vi "I2C WriteRead Data.vi"(5 "Address":T2 format="%02x", 6 "NoStop (F)":bool, 7 "I2C #":T1=-1, 8 "error in (no error)":errorcluster, 9 "Len":u8, 10 "Write Data":string, 11 "Session in":refnum<class "Session.lvclass">) -> (0 "error out":errorcluster, 1 "Read Data":string, 3 "Session out":refnum<class "Session.lvclass">)   [LabVIEW 2020, in "CTI.lvlib" / "Session.lvclass"]
uses:
  Session.lvclass
  I2C Address.ctl
  I2C Number.ctl
  DeviceComms/DeviceComms.lvclass
  CTI.lvlib
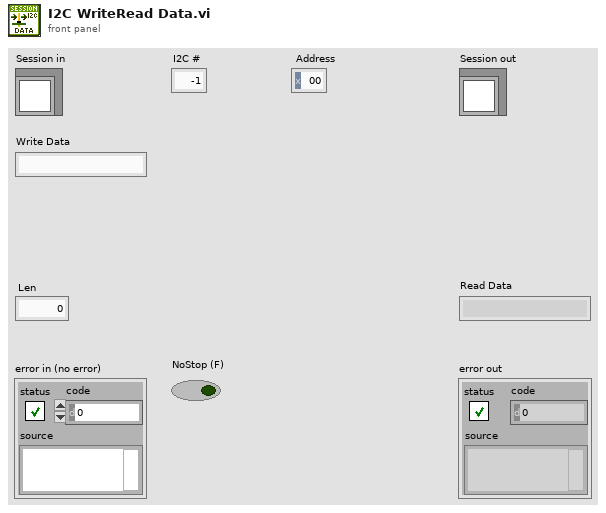
[diagram p1: front panel]
types:
  T1 = typedef "CTI.lvlib/I2C Number.ctl" = i8
  T2 = typedef "CTI.lvlib/I2C Address.ctl" = u8
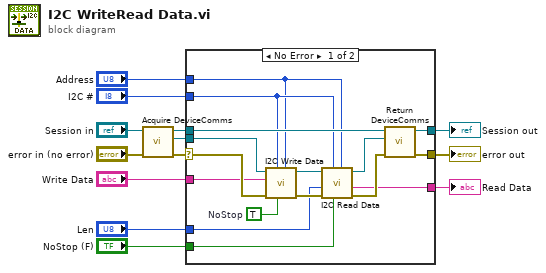
[diagram p0: block diagram]
diagram:
  n1 = call "Acquire DeviceComms.vi"("error in (no error)"="error in (no error)", "Session in"="Session in") -> ("error out"=w12:errorcluster, "DeviceComms"=w11:refnum<class "DeviceComms.lvclass">, "Session out"=w13:refnum<class "Session.lvclass">)  [unwired: 7 in]
  n2 = case shown="No Error" w12 {
    selector: w12 -> [w28 w31]
    tunnel: w13 -> [w27 w30]
    tunnel: w11 -> [w29 _]
    tunnel: [w25 w30] -> w2
    tunnel: [w24 w31] -> w3
    tunnel: "I2C #" -> [w19 _]
    tunnel: "Write Data" -> [w23 _]
    tunnel: "Address" -> [w18 _]
    tunnel: "Len" -> [w17 _]
    tunnel: "NoStop (F)" -> [w16 _]
    tunnel: [w14 _] -> w1
    frame No Error {
      w15 = TRUE  # NoStop
      n3 = call-dynamic "I2C Write Data.vi"("Address"=w18, "NoStop (F)"=w15, "I2C #"=w19, "error in (no error)"=w28, "Data"=w23, "DeviceComms in"=w29) -> ("error out"=w26:errorcluster, "DeviceComms out"=w21:refnum<class "DeviceComms.lvclass">)  [unwired: 4 in]
      n4 = call-dynamic "I2C Read Data.vi"("Address"=w18, "NoStop (F)"=w16, "I2C #"=w19, "error in (no error)"=w26, "Len"=w17, "DeviceComms in"=w21) -> ("error out"=w22:errorcluster, "Data"=w14:string, "DeviceComms out"=w20:refnum<class "DeviceComms.lvclass">)  [unwired: 3 in]
      n5 = call "Return DeviceComms.vi"("error in (no error)"=w22, "DeviceComms"=w20, "Session in"=w27) -> ("error out"=w24:errorcluster, "Session out"=w25:refnum<class "Session.lvclass">)  [unwired: 7 in]
    }
    frame Error {
    }
  }
  "error out" <- w3
  "Session out" <- w2
  "Read Data" <- w1
